vi "InOutVol2Points.vi"(9 "out_vol":dbl, 10 "in_vol":dbl, 11 "tank":T1) -> (0 "remainder_out_vol":dbl, 1 "out_points":i32, 2 "remainder_in_vol":dbl, 3 "in_points":i32)   [LabVIEW 2020]
uses:
  TankResolution.ctl
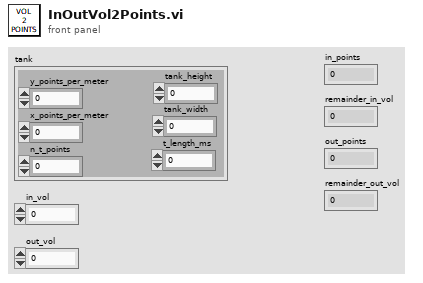
[diagram p1: front panel]
types:
  T1 = typedef "TankResolution.ctl" = cluster{"y_points_per_meter":i32, "x_points_per_meter":i32, "n_t_points":i32, "tank_height":dbl, "tank_width":dbl, "t_length_ms":u32}
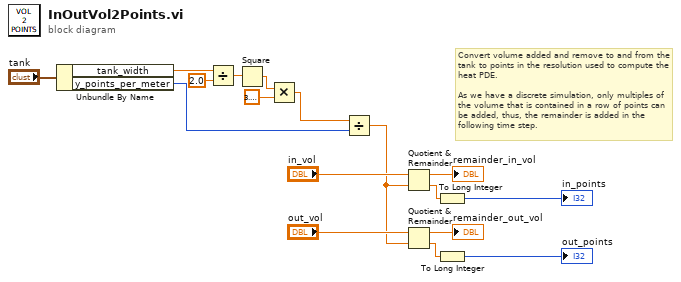
[diagram p0: block diagram]
diagram:
  # "Convert volume added and remove to and from the tank to points in the resolution used to compute the heat PDE.\n\nAs we have a discrete simulation, only multiples of the volume that is contained in a row of points can be added, thus, the remainder is added in the following time step."
  n1 = Unbundle By Name("tank") -> ("tank_width"=w5:dbl, "y_points_per_meter"=w14:i32)
  n2 = Divide(x=w5, y=2.0) -> (x/y=w6:dbl)
  n3 = Square(x=w6) -> (x^2=w3:dbl)
  n4 = Multiply(x=w3, y=3.141592653589793) -> (x*y=w1:dbl)
  n5 = Divide(x=w1, y=w14) -> (x/y=w10:dbl)
  n6 = Quotient & Remainder(x="in_vol", y=w10) -> (x-y*floor(x/y)=→"remainder_in_vol":dbl, floor(x/y)=w12:dbl)
  n7 = Quotient & Remainder(x="out_vol", y=w10) -> (x-y*floor(x/y)=→"remainder_out_vol":dbl, floor(x/y)=w13:dbl)
  n8 = To Long Integer(number=w12) -> (32bit integer=→"in_points":i32)
  n9 = To Long Integer(number=w13) -> (32bit integer=→"out_points":i32)
